vi "Right Buttons.vi"(7 "Message type":string, 8 "error constant":errorcluster, 9 "Input":string, 10 "reference":refnum<vi>) -> (0 "error out":errorcluster, 2 "Action":T1, 4 "Pin Out":string, 5 "Msg":string)   [LabVIEW 2019, in "SubVI.lvlib"]
doc: "Performs Functions Set by right buttons on the UI"
uses:
  controls/ATM Action.ctl
  controls/Message Type.ctl
  SubVIs/SubVI.lvlib
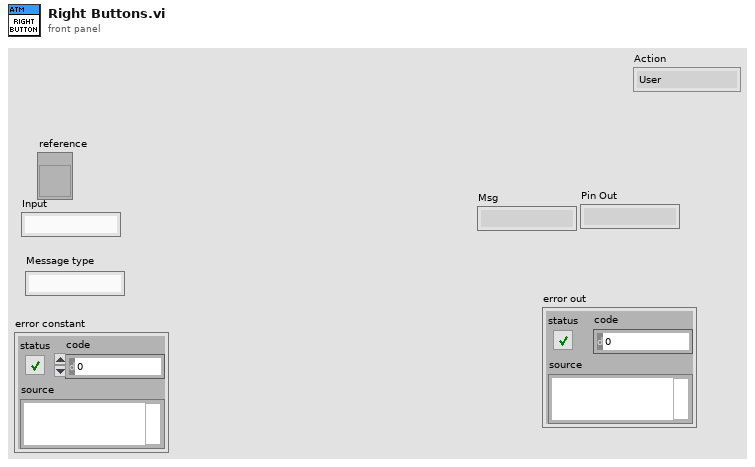
[diagram p1: front panel]
types:
  T1 = typedef "ATM Action.ctl" = enum16{"User", "Deposit", "Withdraw"}
  T2 = typedef "Message Type.ctl" = enum16{"Main Menu", "Balance", "Withdrawal Complete", "Deposit Complete", "Welcome", "Account", "Session", "Deposit", "Withdraw", "Failed"}
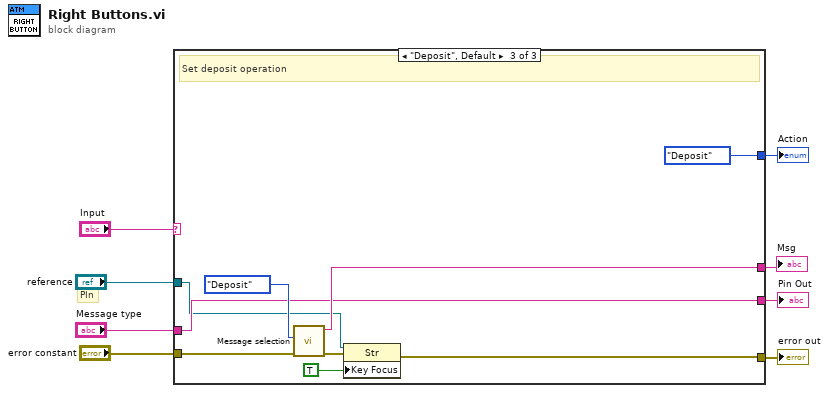
[diagram p0: block diagram]
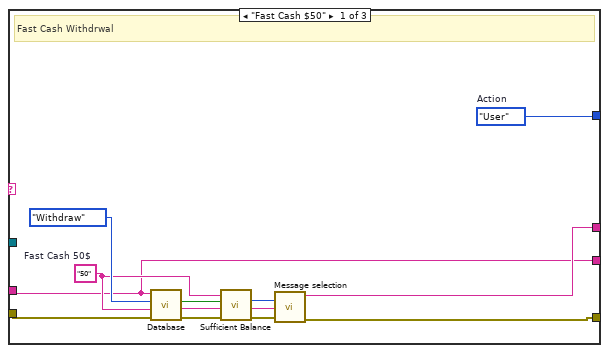
[diagram p2: hidden frame]
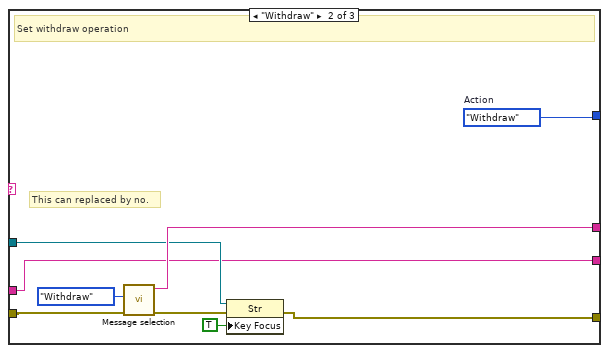
[diagram p3: hidden frame]
diagram:
  # "PIn"
  n1 = case shown="\"Deposit\", Default" "Input" {
    tunnel: "error constant" -> [w19 w27 w36]
    tunnel: [w20 w29 w38] -> w5
    tunnel: [w21 w28 ATM_Action."Deposit" ("Action")] -> w2
    tunnel: [w17 w25 w33] -> w4
    tunnel: "Message type" -> [w9 w22 w32]
    tunnel: "reference" -> [_ w23 w31]
    tunnel: [w9 w22 w32] -> w3
    frame "Fast Cash $50" {
      w21 = ATM_Action."User"  # Action
      w15 = "50"  # Fast Cash 50$
      # "Fast Cash Withdrwal"
      n2 = call "Database.vi"("error in"=w19, "Money In"=w15, "Action"=ATM_Action."Withdraw", "User Input"=w9) -> ("error out"=w14:errorcluster, "Money Out"=w12:string, "Done"=w16:bool)  [unwired: 4 in, 1 out]
      n3 = call "Sufficient Balance.vi"("error in (no error)"=w14, "Money In"=w12, "Valid"=w16, "Fast Cash 50$"=w15) -> ("error out"=w13:errorcluster, "Money Out"=w11:string, "state"=w10:T2)  [unwired: 4 in, 1 out]
      n4 = call "Message selection.vi"("error in (no error)"=w13, "Amount"=w11, "state"=w10) -> ("error out"=w20:errorcluster, "Msg"=w17:string)  [unwired: 7 in]
    }
    frame "Withdraw" {
      w28 = ATM_Action."Withdraw"  # Action
      # "This can replaced by no."
      # "Set withdraw operation"
      n5 = call "Message selection.vi"("error in (no error)"=w27, "state"=Message_Type."Withdraw") -> ("error out"=w24:errorcluster, "Msg"=w25:string)  [unwired: 8 in]
      n6 = property on="Property Node" class="Str"(reference=w23, error in=w24, "Key Focus"=TRUE) -> (error out=w29:errorcluster)  [unwired: 1 out]
    }
    frame "Deposit", Default {
      # "Set deposit operation"
      n7 = call "Message selection.vi"("error in (no error)"=w36, "state"=Message_Type."Deposit") -> ("error out"=w35:errorcluster, "Msg"=w33:string)  [unwired: 8 in]
      n8 = property on="Property Node" class="Str"(reference=w31, error in=w35, "Key Focus"=TRUE) -> (error out=w38:errorcluster)  [unwired: 1 out]
    }
  }
  "error out" <- w5
  "Msg" <- w4
  "Pin Out" <- w3
  "Action" <- w2
